vi "Big_LED_control.vi"() -> ()   [LabVIEW 2018]
uses:
  <instrlib>/niDCPower/nidcpower.llb/niDCPower Measurement Type.ctl
  <vilib>/Instr/_visa.llb/VISA Configure Serial Port (Instr).vi
  <instrlib>/niDMM/nidmm.llb/niDMM Function.ctl
  <instrlib>/niDMM/nidmm.llb/niDMM Resolution in Digits.ctl
  <instrlib>/niDMM/nidmm.llb/niDMM Configure Measurement Digits.vi
panel:
  in  "Tab Control":enum32{"Рабочая область", "Служебная область"}(tab)
  out "Тип индикатора":string
  in  "Питание":bool
  in  "Стоп":bool
  in  "Resource Name":refnum<k15>="PXI1Slot2" caption="Источник питания"
  in  "Амперметр":refnum<k15>="PXI1Slot5" caption="NI DMM 1"
  in  "V_MB, V":dbl=6.0 caption="voltage level" format="%_6p"
  in  "curlim_V_MB, A":dbl=0.3 caption="current limit" format="%_6p"
  in  "curlim_V_RESERVE, A":dbl=0.1 caption="current limit" format="%_6p"
  out "currentmes_V_MB, A":dbl caption="measurement" format="%_6g"
  out "currentmes_V_RESERVE, A":dbl caption="measurement" format="%_6g"
  in  "V_RESERVE, V":dbl caption="voltage level" format="%_6p"
  out "chart_2":dbl(graph)=8.556104343922883e-07
  out "chart_0":dbl(graph)=5.42616690347781e-05 caption="Waveform Chart 5"
  in  "curlim_V_LED, A":dbl=0.03 caption="current limit" format="%_6p"
  in  "V_LED, V":dbl=2.000000000000001 caption="voltage level" format="%_6p"
  out "chart_1":dbl(graph)=2.456762028615791e-06 caption="Waveform Chart 5"
  out "currentmes_V_LED, A":dbl caption="measurement" format="%_6g"
  in  "NI DMM 1 Current Range 3":string(combo)="0,1" caption="Range"
  out "Current, А":dbl=1.3612861948786303e-08 format="%.5f"
  in  "NI DMM 1 units 3":string(combo)="1000" caption="Units"
  out "NI DMM 1 Current Char 3":dbl(graph)=0.013612861948786303
  out "NI DMM 1 Current 3":dbl caption="Current" format="%_6g"
  in  "Arduino":refnum<visa-resource-name>="COM14"
  in  "Сегменты":bool[](array[boolean])=[FALSE, FALSE, FALSE, FALSE, FALSE, FALSE, FALSE, FALSE, FALSE, FALSE]
  in  "Вольтметр":refnum<k15>="PXI1Slot5" caption="NI DMM 1"
  in  "NI DMM 1 Voltage Range 4":string(combo)="0,1" caption="Range"
  out "NI DMM 1 Voltage Char 4":dbl(graph)=0.013612861948786303
  out "Voltage, V":dbl=1.3612861948786303e-08 format="%.5f"
  in  "NI DMM 1 units 4":string(combo)="1000" caption="Units"
  out "NI DMM 1 Voltage 4":dbl caption="Voltage" format="%_6g"
  out "Разряд":dbl
  out "+/-":bool
  in  "Записать":bool
  in  "Command":string="led_on"
  out "Power off":bool
  # "all_off - 0\nall_on - 1"
  # "j"
  # "c"
  # "d"
  # "e"
  # "g"
  # "h"
  # "a"
  # "b"
  # "f"
  # "k"
  # "L"
  # "m"
  # "n"
  # "p"
  # "dp"
  # "необходимо выдерживать 1 с между нажатиями кнопок"
  # "регулировать ток в зависимости от температуры.\nс ростом температуры растет ток.\nпид-регулятор??"
  # "\"опрашивать кнопки не чаще, чем раз в секунду. сейчас кликать можно чаще, они загорятся, но ничего не произойдет\""
  # "автоматизировать подбор напряжения по известному максимальному напряжению и току. ОС по току сегмента"
  # "регклировка суммарного тока через инлдикатор"
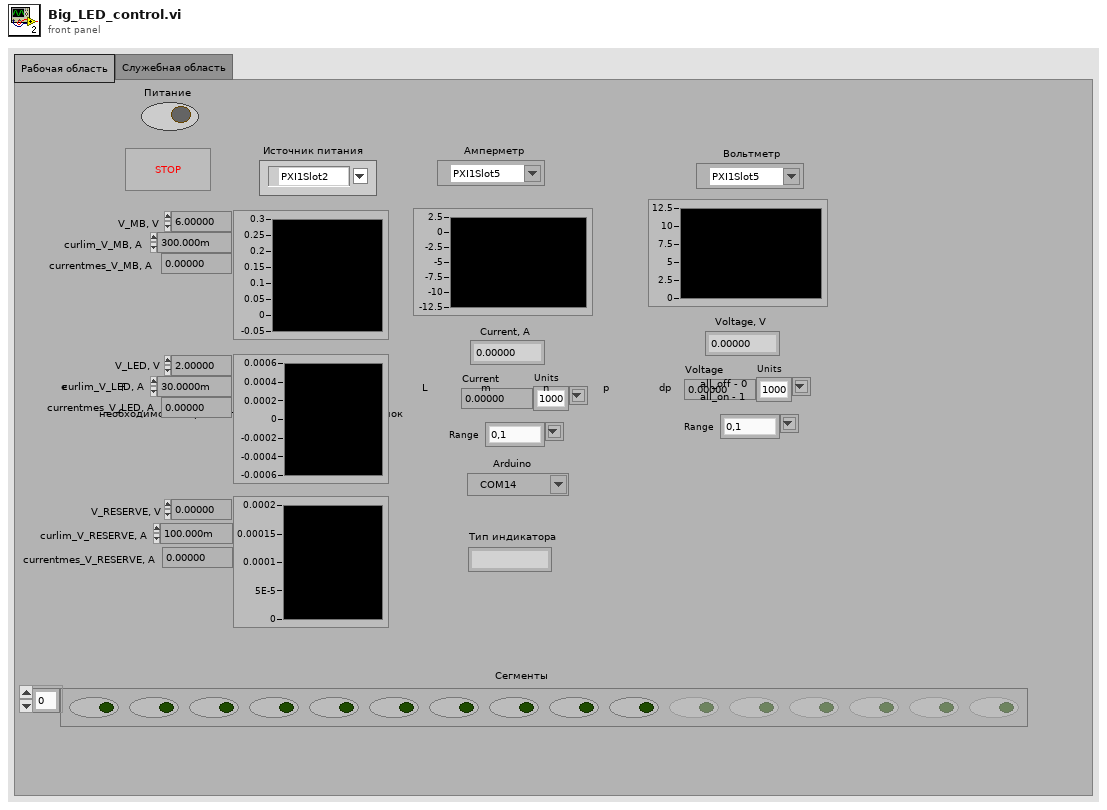
[diagram p1: front panel]
types:
  T1 = typedef "niDMM Function.ctl" = enum16{"DC Volts", "AC Volts", "DC Current", "AC Current", "2-wire Resistance", "4-wire Resistance", "Diode", "Frequency", "Period", "AC Volts DC Coupled", "Capacitance", "Inductance", "Temperature"}
  T2 = typedef "niDMM Resolution in Digits.ctl" = dbl
  T3 = typedef "niDCPower Measurement Type.ctl" = i32
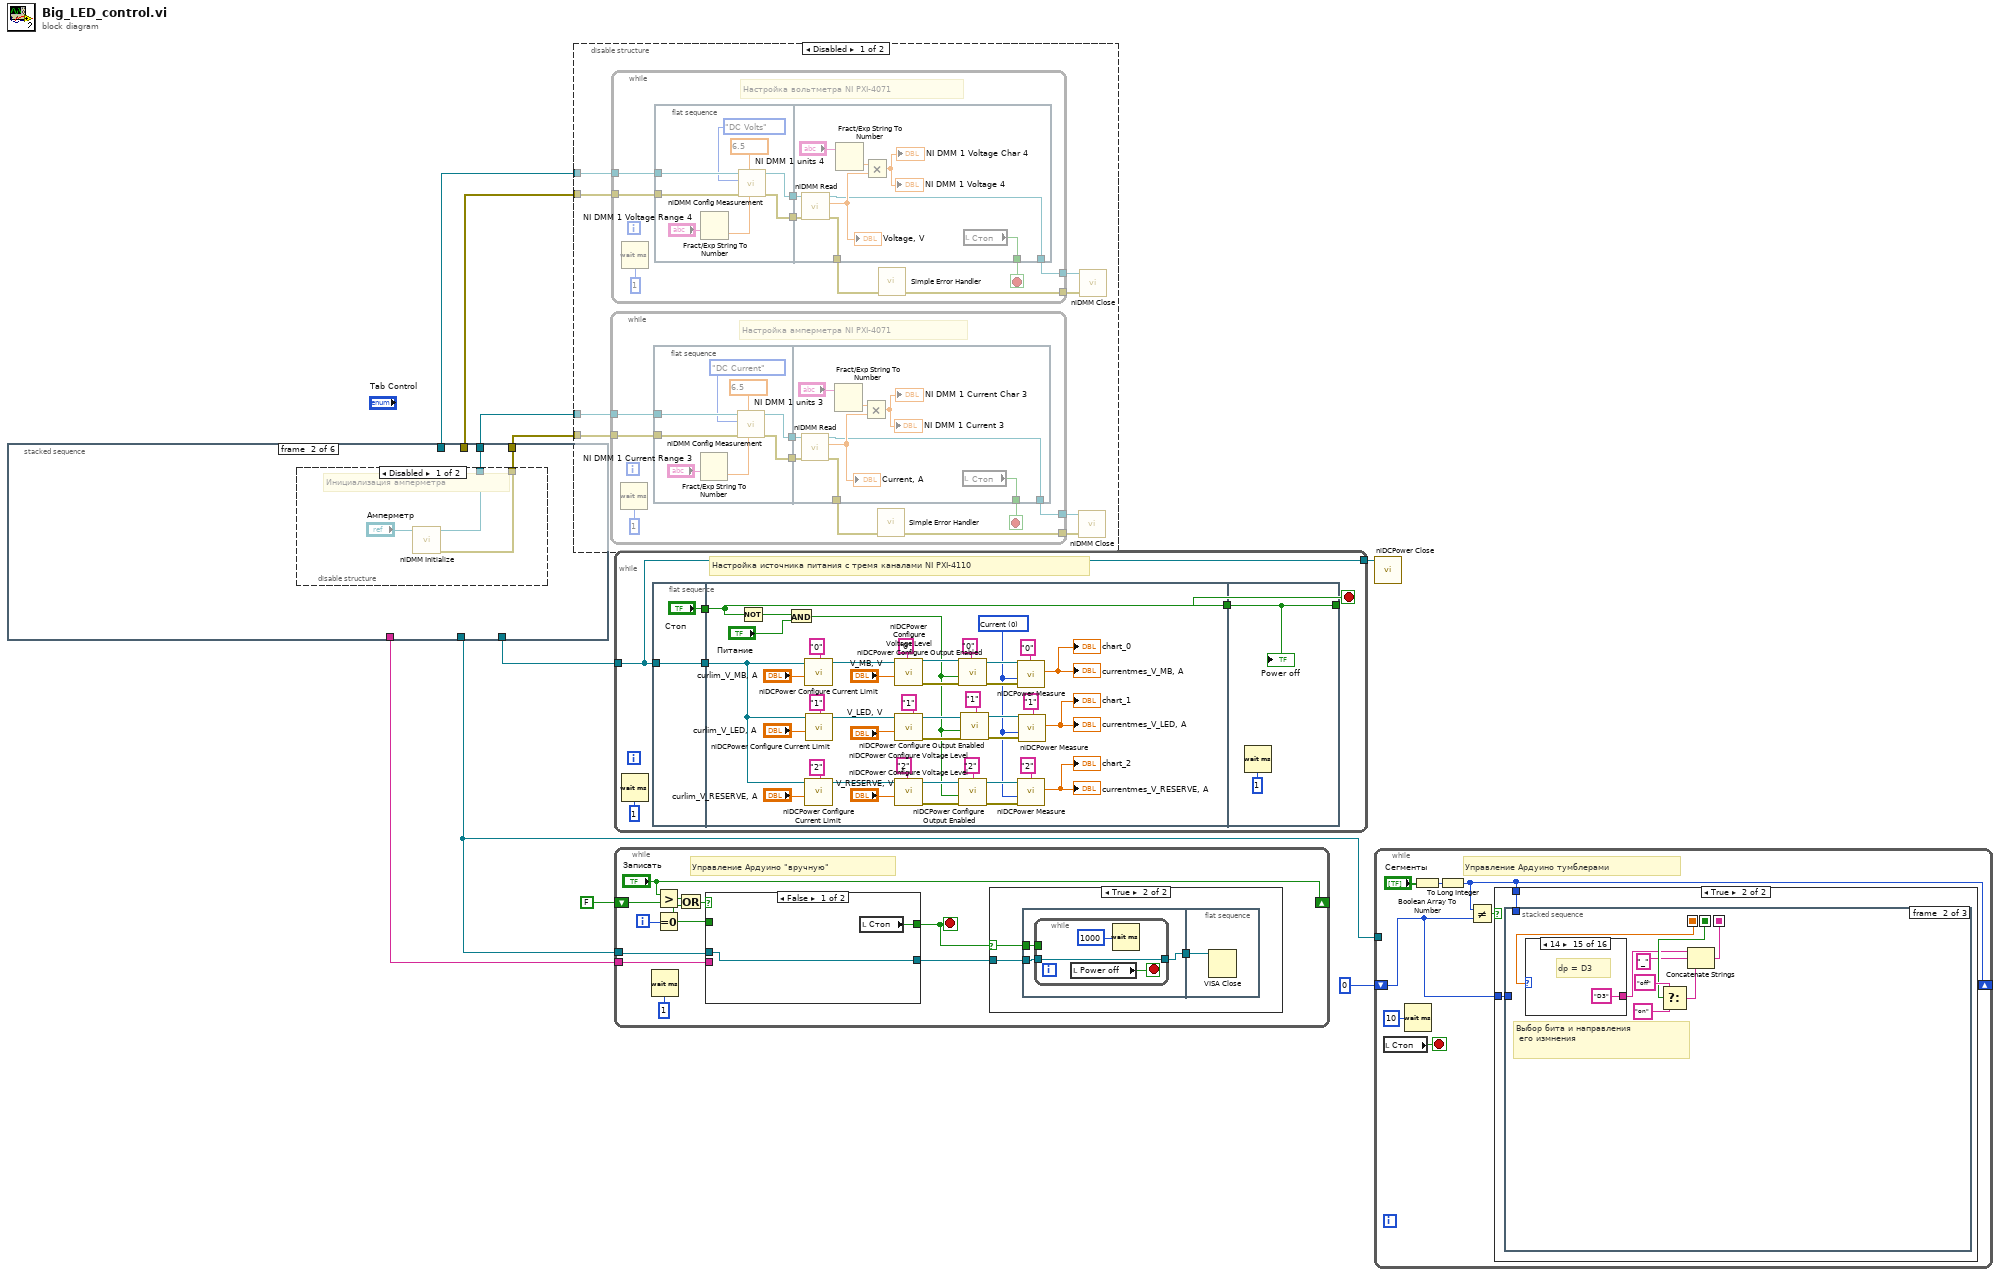
[diagram p0: block diagram]
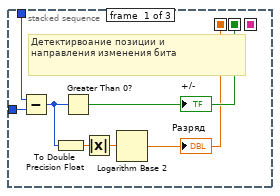
[diagram p4: hidden frame]
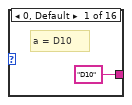
[diagram p5: hidden frame]
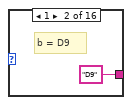
[diagram p6: hidden frame]
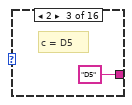
[diagram p7: hidden frame]
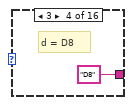
[diagram p8: hidden frame]
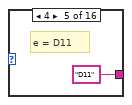
[diagram p9: hidden frame]
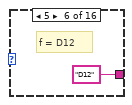
[diagram p10: hidden frame]
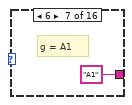
[diagram p11: hidden frame]
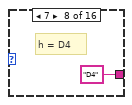
[diagram p12: hidden frame]
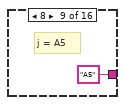
[diagram p13: hidden frame]
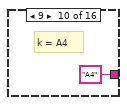
[diagram p14: hidden frame]
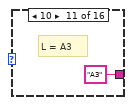
[diagram p15: hidden frame]
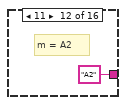
[diagram p16: hidden frame]
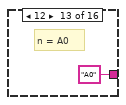
[diagram p17: hidden frame]
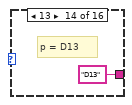
[diagram p18: hidden frame]
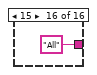
[diagram p19: hidden frame]
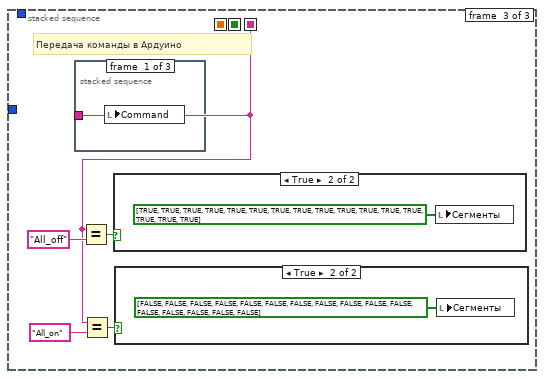
[diagram p20: hidden frame]
diagram:
  n1 = stacked-sequence {
    tunnel: [_ _ _ w27 _ _] -> w7
    tunnel: [_ w16 _ _ _ _] -> w10
    tunnel: [_ w15 _ _ _ _] -> w9
    tunnel: [_ _ _ _ w31 _] -> w4
    tunnel: [_ _ _ _ _ w34] -> w3
    tunnel: [_ _ w21 _ _ _] -> w2
    tunnel: [_ _ w20 _ _ _] -> w1
    frame #0 {
      w13 = 0.0 ("currentmes_2")
      w12 = FALSE ("Стоп")
      # "Обнуление переменных"
      n2 = local write "Питание"(w12) -> ()
      n3 = local write "Стоп"(w12) -> ()
      n4 = local write "+/-"(w12) -> ()
      n5 = local write "Сегменты"(bool[] [FALSE, FALSE, FALSE, FALSE, FALSE, FALSE, FALSE, FALSE, FALSE, FALSE, FALSE, FALSE, FALSE, FALSE, FALSE, FALSE, FALSE, FALSE] ("Сегменты")) -> ()
      n6 = local write "currentmes_V_MB, A"(w13) -> ()
      n7 = local write "currentmes_V_LED, A"(w13) -> ()
      n8 = local write "currentmes_V_RESERVE, A"(w13) -> ()
      n9 = local write "NI DMM 1 Current 3"(w13) -> ()
      n10 = local write "Разряд"(w13) -> ()
      n11 = local write "Command"("zero" ("Command 2")) -> ()
    }
    frame #1 {
      n12 = disable-structure shown="Disabled" {
        disable-tunnel: [w19 _] -> w16
        disable-tunnel: [w18 _] -> w15
        frame Disabled {
          # "Инициализация амперметра"
          n13 = call <instrlib>:"niDMM Initialize.vi"("Instrument Descriptor"="Амперметр") -> ("error out"=w19:errorcluster, "instrument handle out"=w18:refnum<k15>)  [unwired: 9 in]
        }
        frame Enabled {
        }
      }
    }
    frame #2 {
      n14 = disable-structure shown="Disabled" {
        disable-tunnel: [w24 _] -> w21
        disable-tunnel: [w23 _] -> w20
        frame Disabled {
          # "Инициализация вольтметра"
          n15 = call <instrlib>:"niDMM Initialize.vi"("Instrument Descriptor"="Вольтметр") -> ("error out"=w23:errorcluster, "instrument handle out"=w24:refnum<k15>)  [unwired: 9 in]
        }
        frame Enabled {
        }
      }
    }
    frame #3 {
      # "Инициализация источника питания"
      n16 = call <instrlib>:"niDCPower Initialize.vi"("resource name"="Resource Name") -> ("error out"=w26:errorcluster, "instrument handle out"=w28:refnum<k15>)  [unwired: 3 in, 6 out]
      n17 = call <instrlib>:"niDCPower Configure Voltage Level.vi"("error in (no error)"=w26, "voltage level"=0.0, "channel name"="0,1,2", "instrument handle"=w28) -> ("instrument handle out"=w27:refnum<k15>)  [unwired: 6 in, 1 out]
    }
    frame #4 {
      # "Инициализация Ардуино"
      n18 = call-poly "VISA Configure Serial Port"("VISA resource name"="Arduino", "baud rate (9600)"=u32 9600) -> ("VISA resource name out"=w31:refnum<visa-resource-name>)  [unwired: 12 in, 1 out]
    }
    frame #5 {
      # "Всплывающее окно\nкакой индикатор?\nОА/ОК"
      n19 = call "Begin.vi"() -> ("String"=w34:string)  [unwired: 8 in]
      "Тип индикатора" <- w34
      n20 = local write "Command"(w34) -> ()
    }
  }
  n21 = disable-structure shown="Disabled" {
    disable-tunnel: w10 -> [w42 _]
    disable-tunnel: w9 -> [w41 _]
    disable-tunnel: w2 -> [w40 _]
    disable-tunnel: w1 -> [w39 _]
    frame Disabled {
      n22 = while {
        tunnel: [w49] -> w35
        tunnel: w41 -> [w47]
        tunnel: w42 -> [w46]
        tunnel: [w43] -> w36
        stop <- w45 stop-if-true
        # "Настройка амперметра NI PXI-4071"
        n23 = Wait (ms)(milliseconds to wait=u32 1) -> ()  [unwired: 1 out]
        n24 = flat-sequence {
          tunnel: [w56] -> w51
          tunnel: w47 -> [w54]
          tunnel: w46 -> [w58]
          tunnel: [w55] -> w50
          tunnel: w51 -> [w64]
          tunnel: w50 -> [w67]
          tunnel: [w62] -> w45
          tunnel: [w61] -> w43
          tunnel: [w60] -> w44
          frame #0 {
            w52 = T2 6.5 items=["3 1/2"=3.5, "4 1/2"=4.5, "5 1/2"=5.5, "6 1/2"=6.5, "7 1/2"=7.5] ("Resolution in Digits")
            n25 = Fract/Exp String To Number(string="NI DMM 1 Current Range 3") -> (number=w57:dbl)  [unwired: 3 in, 1 out]
            n26 = call-poly <instrlib>:"niDMM Config Measurement.vi"("Range"=w57, "Resolution in Digits"=w52, "error in (no error)"=w58, "Function"=niDMM_Function."DC Current" ("Measurement Type"), "instrument handle"=w54) -> ("error out"=w55:errorcluster, "instrument handle out"=w56:refnum<k15>)  [unwired: 5 in]
          }
          frame #1 {
            n27 = call <instrlib>:"niDMM Read.vi"("error in (no error)"=w67, "instrument handle"=w64) -> ("error out"=w60:errorcluster, "Measurement"=w63:dbl, "instrument handle out"=w61:refnum<k15>)  [unwired: 7 in]
            "Current, А" <- w63
            n28 = Fract/Exp String To Number(string="NI DMM 1 units 3") -> (number=w65:dbl)  [unwired: 3 in, 1 out]
            n29 = Multiply(x=w65, y=w63) -> (x*y=→"NI DMM 1 Current 3" →"NI DMM 1 Current Char 3":dbl)
            n30 = local read "Стоп"() -> (w62:bool)
          }
        }
        n31 = call <vilib>:"Simple Error Handler.vi"("error in (no error)"=w44) -> ("error out"=w49:errorcluster)  [unwired: 1 in, 7 out]
      }
      n32 = while {
        tunnel: [w75] -> w37
        tunnel: w40 -> [w73]
        tunnel: w39 -> [w72]
        tunnel: [w69] -> w38
        stop <- w71 stop-if-true
        # "Настройка вольтметра NI PXI-4071"
        n33 = Wait (ms)(milliseconds to wait=u32 1) -> ()  [unwired: 1 out]
        n34 = flat-sequence {
          tunnel: [w82] -> w77
          tunnel: w73 -> [w80]
          tunnel: w72 -> [w84]
          tunnel: [w81] -> w76
          tunnel: w77 -> [w90]
          tunnel: w76 -> [w93]
          tunnel: [w88] -> w71
          tunnel: [w87] -> w69
          tunnel: [w86] -> w70
          frame #0 {
            w78 = T2 6.5 items=["3 1/2"=3.5, "4 1/2"=4.5, "5 1/2"=5.5, "6 1/2"=6.5, "7 1/2"=7.5] ("Resolution in Digits")
            n35 = Fract/Exp String To Number(string="NI DMM 1 Voltage Range 4") -> (number=w83:dbl)  [unwired: 3 in, 1 out]
            n36 = call-poly <instrlib>:"niDMM Config Measurement.vi"("Range"=w83, "Resolution in Digits"=w78, "error in (no error)"=w84, "Function"=niDMM_Function."DC Volts" ("Measurement Type"), "instrument handle"=w80) -> ("error out"=w81:errorcluster, "instrument handle out"=w82:refnum<k15>)  [unwired: 5 in]
          }
          frame #1 {
            n37 = call <instrlib>:"niDMM Read.vi"("error in (no error)"=w93, "instrument handle"=w90) -> ("error out"=w86:errorcluster, "Measurement"=w89:dbl, "instrument handle out"=w87:refnum<k15>)  [unwired: 7 in]
            "Voltage, V" <- w89
            n38 = Fract/Exp String To Number(string="NI DMM 1 units 4") -> (number=w91:dbl)  [unwired: 3 in, 1 out]
            n39 = Multiply(x=w91, y=w89) -> (x*y=→"NI DMM 1 Voltage 4" →"NI DMM 1 Voltage Char 4":dbl)
            n40 = local read "Стоп"() -> (w88:bool)
          }
        }
        n41 = call <vilib>:"Simple Error Handler.vi"("error in (no error)"=w70) -> ("error out"=w75:errorcluster)  [unwired: 1 in, 7 out]
      }
      n42 = call <instrlib>:"niDMM Close.vi"("error in (no error)"=w35, "instrument handle"=w36) -> ()  [unwired: 9 in, 1 out]
      n43 = call <instrlib>:"niDMM Close.vi"("error in (no error)"=w37, "instrument handle"=w38) -> ()  [unwired: 9 in, 1 out]
    }
    frame Enabled {
    }
  }
  n44 = while {
    tunnel: w7 -> [w96]
    tunnel: [w96] -> w6
    stop <- w97 stop-if-true
    # "Настройка источника питания с тремя каналами NI PXI-4110"
    n45 = Wait (ms)(milliseconds to wait=u32 1) -> ()  [unwired: 1 out]
    n46 = flat-sequence {
      tunnel: w96 -> [w102]
      tunnel: [w102] -> w99
      tunnel: ["Стоп"] -> w98
      tunnel: w99 -> [w110]
      tunnel: w98 -> [w144]
      tunnel: [w144] -> w95
      tunnel: [w146] -> w97
      tunnel: w95 -> [w146]
      frame #0 {
      }
      frame #1 {
        w109 = T3 0 items=["Current", "Voltage"] ("measurement type")
        n47 = Not(x=w144) -> (.not. x?=w143:bool)
        n48 = And(x=w143, y="Питание") -> (x .and. y?=w105:bool)
        n49 = call <instrlib>:"niDCPower Configure Current Limit.vi"("current limit"="curlim_V_MB, A", "channel name"="0", "instrument handle"=w110) -> ("instrument handle out"=w129:refnum<k15>)  [unwired: 7 in, 1 out]
        n50 = call <instrlib>:"niDCPower Configure Current Limit.vi"("current limit"="curlim_V_RESERVE, A", "channel name"="2", "instrument handle"=w110) -> ("instrument handle out"=w128:refnum<k15>)  [unwired: 7 in, 1 out]
        n51 = call <instrlib>:"niDCPower Configure Current Limit.vi"("current limit"="curlim_V_LED, A", "channel name"="1", "instrument handle"=w110) -> ("instrument handle out"=w137:refnum<k15>)  [unwired: 7 in, 1 out]
        n52 = call <instrlib>:"niDCPower Configure Voltage Level.vi"("voltage level"="V_MB, V", "channel name"="0", "instrument handle"=w129) -> ("error out"=w134:errorcluster, "instrument handle out"=w131:refnum<k15>)  [unwired: 7 in]
        n53 = call <instrlib>:"niDCPower Configure Voltage Level.vi"("voltage level"="V_LED, V", "channel name"="1", "instrument handle"=w137) -> ("error out"=w140:errorcluster, "instrument handle out"=w138:refnum<k15>)  [unwired: 7 in]
        n54 = call <instrlib>:"niDCPower Configure Voltage Level.vi"("voltage level"="V_RESERVE, V", "channel name"="2", "instrument handle"=w128) -> ("error out"=w133:errorcluster, "instrument handle out"=w132:refnum<k15>)  [unwired: 7 in]
        n55 = call <instrlib>:"niDCPower Configure Output Enabled.vi"("error in (no error)"=w134, "output enabled"=w105, "channel name"="0", "instrument handle"=w131) -> ("error out"=w124:errorcluster, "instrument handle out"=w125:refnum<k15>)  [unwired: 6 in]
        n56 = call <instrlib>:"niDCPower Configure Output Enabled.vi"("error in (no error)"=w133, "output enabled"=w105, "channel name"="2", "instrument handle"=w132) -> ("error out"=w123:errorcluster, "instrument handle out"=w122:refnum<k15>)  [unwired: 6 in]
        n57 = call <instrlib>:"niDCPower Configure Output Enabled.vi"("error in (no error)"=w140, "output enabled"=w105, "channel name"="1", "instrument handle"=w138) -> ("error out"=w141:errorcluster, "instrument handle out"=w139:refnum<k15>)  [unwired: 6 in]
        n58 = call <instrlib>:"niDCPower Measure.vi"("error in (no error)"=w124, "measurement type"=w109, "channel name"="0", "instrument handle"=w125) -> ("measurement"=→"currentmes_V_MB, A" →"chart_0":dbl)  [unwired: 5 in, 2 out]
        n59 = call <instrlib>:"niDCPower Measure.vi"("error in (no error)"=w123, "measurement type"=w109, "channel name"="2", "instrument handle"=w122) -> ("measurement"=→"currentmes_V_RESERVE, A" →"chart_2":dbl)  [unwired: 5 in, 2 out]
        n60 = call <instrlib>:"niDCPower Measure.vi"("error in (no error)"=w141, "measurement type"=w109, "channel name"="1", "instrument handle"=w139) -> ("measurement"=→"chart_1" →"currentmes_V_LED, A":dbl)  [unwired: 5 in, 2 out]
      }
      frame #2 {
        n61 = Wait (ms)(milliseconds to wait=u32 1) -> ()  [unwired: 1 out]
        "Power off" <- w146
      }
    }
  }
  n62 = while {
    tunnel: w4 -> [w154]
    shift-right: ["Записать"] -> _
    shift-left: FALSE ("Записать") -> [w156]
    tunnel: w3 -> [w152]
    i -> [w153]
    stop <- w148 stop-if-true
    # "Управление Ардуино \"вручную\""
    n63 = Wait (ms)(milliseconds to wait=u32 1) -> ()  [unwired: 1 out]
    n64 = Greater?(x="Записать", y=w156) -> (0:w150:bool)
    n65 = Equal To 0?(x=w153) -> (x = 0?=w149:bool)
    n66 = Or(x=w150, y=w149) -> (x .or. y?=w151:bool)
    n67 = case shown="False" w151 {
      tunnel: w154 -> [w168 w173]
      tunnel: [w169 w172] -> w148
      tunnel: w152 -> [_ _]
      tunnel: w149 -> [_ _]
      tunnel: [w168 w170] -> w147
      frame False {
        n68 = local read "Стоп"() -> (w169:bool)
      }
      frame True {
        n69 = VISA Write(VISA resource name=w173, write buffer="Command") -> (VISA resource name out=w170:refnum<visa-resource-name>)  [unwired: 1 in, 2 out]
        n70 = local read "Стоп"() -> (w172:bool)
      }
    }
    n71 = case shown="True" w148 {
      selector: w148 -> [_ w158]
      tunnel: w147 -> [_ w160]
      frame False {
      }
      frame True {
        n72 = flat-sequence {
          tunnel: w160 -> [w163]
          tunnel: [w162] -> w159
          tunnel: w158 -> [w161]
          tunnel: w159 -> [w167]
          frame #0 {
            n73 = while {
              tunnel: w163 -> [w166]
              tunnel: [w166] -> w162
              tunnel: w161 -> [_]
              stop <- w164 stop-if-true
              n74 = local read "Power off"() -> (w164:bool)
              n75 = Wait (ms)(milliseconds to wait=u32 1000) -> ()  [unwired: 1 out]
            }
          }
          frame #1 {
            n76 = VISA Close(VISA resource name=w167) -> ()  [unwired: 1 in, 1 out]
          }
        }
      }
    }
  }
  n77 = call <instrlib>:"niDCPower Close.vi"("instrument handle"=w6) -> ()  [unwired: 10 in, 1 out]
  n78 = while {
    shift-right: [w175] -> _
    shift-left: i16 0 -> [w176]
    tunnel: w4 -> [_]
    stop <- w180 stop-if-true
    # "Управление Ардуино тумблерами"
    n79 = local read "Стоп"() -> (w180:bool)
    n80 = Wait (ms)(milliseconds to wait=u32 10 ("millisecond timer value")) -> ()  [unwired: 1 out]
    n81 = Boolean Array To Number(Boolean array="Сегменты") -> (number=w174:u32)
    n82 = To Long Integer(number=w174) -> (32bit integer=w175:i32)
    n83 = Not Equal?(x=w175, y=w176) -> (x != y?=w177:bool)
    n84 = case shown="True" w177 {
      tunnel: w175 -> [_ w181]
      tunnel: w176 -> [_ w182]
      frame False {
      }
      frame True {
        n85 = stacked-sequence {
          seq-local: [w185 _ _] -> [_ w195 _]
          seq-local: [w183 _ _] -> [_ w190 _]
          seq-local: [_ w191 _] -> [_ _ w215]
          tunnel: w181 -> [w187 _ _]
          tunnel: w182 -> [w186 _ _]
          frame #0 {
            # "Детектирвоание позиции и\nнаправления изменения бита"
            n86 = Subtract(x=w187, y=w186) -> (x-y=w188:i32)
            n87 = To Double Precision Float(number=w188) -> (double precision float=w189:dbl)
            n88 = Greater Than 0?(x=w188) -> (x > 0?=w185:bool)
            "+/-" <- w185
            n89 = Absolute Value(x=w189) -> (abs(x)=w184:dbl)
            n90 = Logarithm Base 2(1:w184) -> (0:w183:dbl)
            "Разряд" <- w183
          }
          frame #1 {
            # "Выбор бита и направления\n его измнения"
            n91 = case shown="14" w190 {
              tunnel: ["D10" "D9" "D5" "D8" "D11" "D12" "A1" "D4" "A5" "A4" "A3" "A2" "A0" "D13" "D3" "All"] -> w193
              frame 0, Default {
                # "a = D10"
              }
              frame 1 {
                # "b = D9"
              }
              frame 2 {
                # "c = D5"
              }
              frame 3 {
                # "d = D8"
              }
              frame 4 {
                # "e = D11"
              }
              frame 5 {
                # "f = D12"
              }
              frame 6 {
                # "g = A1"
              }
              frame 7 {
                # "h = D4"
              }
              frame 8 {
                # "j = A5"
              }
              frame 9 {
                # "k = A4"
              }
              frame 10 {
                # "L = A3"
              }
              frame 11 {
                # "m = A2"
              }
              frame 12 {
                # "n = A0"
              }
              frame 13 {
                # "p = D13"
              }
              frame 14 {
                # "dp = D3"
              }
              frame 15 {
              }
            }
            n92 = Select(t="off", s=w195, f="on") -> (s? t:f=w192:string)
            n93 = Concatenate Strings(w193, "_" ("string"), w192) -> (w191:string)
          }
          frame #2 {
            # "Передача команды в Ардуино"
            n94 = stacked-sequence {
              tunnel: w215 -> [w221 _ _]
              frame #0 {
                n95 = local write "Command"(w221) -> ()
              }
              frame #1 {
                n96 = local write "Записать"(TRUE ("Записать")) -> ()
                n97 = Wait (ms)(milliseconds to wait=u32 1000) -> ()  [unwired: 1 out]
              }
              frame #2 {
                n98 = local write "Записать"(FALSE ("Записать")) -> ()
                n99 = Wait (ms)(milliseconds to wait=u32 1000) -> ()  [unwired: 1 out]
              }
            }
            n100 = Equal?(x=w215, y="All_off") -> (x = y?=w218:bool)
            n101 = Equal?(x=w215, y="All_on") -> (x = y?=w216:bool)
            n102 = case shown="True" w218 {
              frame False {
              }
              frame True {
                n103 = local write "Сегменты"(bool[] [TRUE, TRUE, TRUE, TRUE, TRUE, TRUE, TRUE, TRUE, TRUE, TRUE, TRUE, TRUE, TRUE, TRUE, TRUE, TRUE] ("Сегменты")) -> ()
              }
            }
            n104 = case shown="True" w216 {
              frame False {
              }
              frame True {
                n105 = local write "Сегменты"(bool[] [FALSE, FALSE, FALSE, FALSE, FALSE, FALSE, FALSE, FALSE, FALSE, FALSE, FALSE, FALSE, FALSE, FALSE, FALSE, FALSE] ("Сегменты")) -> ()
              }
            }
          }
        }
      }
    }
  }
